vi "Format Event ID.vi"(6 "Channel (Channel A)":enum16{"Channel A", "Channel B"}(ring), 7 "Event Module # (1)":u32=1 min=1 max=14, 9 "Event Type (None)":T1(ring), 10 "Node In":string) -> (1 "Event ID":string, 2 "Node Out":string)   [LabVIEW 2013, in "Keithley 2600 Series.lvlib"]
doc: "This VI will format a string representing an event module's Event Id for use as an input to several of the Advanced Trigger Model VIs."
uses:
  Keithley 2600 Series.lvlib
panel:
  # "(c) 2008 Keithley Instruments, Inc.  ALL RIGHTS RESERVED."
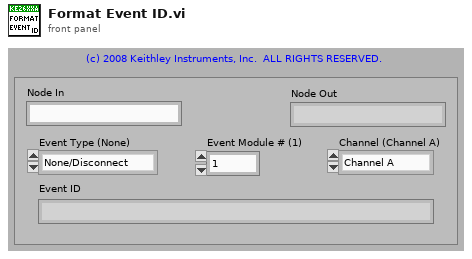
[diagram p1: front panel]
types:
  T1 = enum16{"None/Disconnect", "Digital I/O Trigger", "TSP-Link Trigger", "LAN Trigger", "Blender", "Timer Expired", "Front Panel Trigger", "Software Trigger", "SMU Sweeping", "SMU Armed", "SMU Source Complete", "SMU Measure Complete", "SMU Pulse Complete", "SMU Sweep Complete", "SMU Idle"}
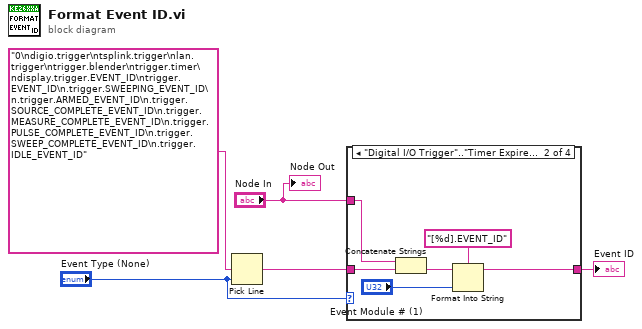
[diagram p0: block diagram]
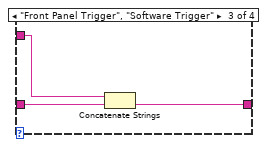
[diagram p3: hidden frame]
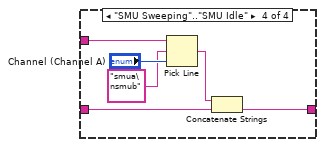
[diagram p4: hidden frame]
diagram:
  n1 = Pick Line(multi-line string="0\ndigio.trigger\ntsplink.trigger\nlan.trigger\ntrigger.blender\ntrigger.timer\ndisplay.trigger.EVENT_ID\ntrigger.EVENT_ID\n.trigger.SWEEPING_EVENT_ID\n.trigger.ARMED_EVENT_ID\n.trigger.SOURCE_COMPLETE_EVENT_ID\n.trigger.MEASURE_COMPLETE_EVENT_ID\n.trigger.PULSE_COMPLETE_EVENT_ID\n.trigger.SWEEP_COMPLETE_EVENT_ID\n.trigger.IDLE_EVENT_ID", line index="Event Type (None)") -> (output string=w3:string)  [unwired: 1 out]
  n2 = case shown="\"Digital I/O Trigger\"..\"Timer Expired\"" "Event Type (None)" {
    tunnel: w3 -> [w6 w9 w14 w19]
    tunnel: [w6 w10 w13 w17] -> w2
    tunnel: "Node In" -> [_ w7 w15 w16]
    frame "None/Disconnect", Default {
    }
    frame "Digital I/O Trigger".."Timer Expired" {
      n3 = Concatenate Strings(w7, w9) -> (w8:string)
      n4 = Format Into String(format string="[%d].EVENT_ID", initial string=w8, "Event Module # (1)") -> (resulting string=w10:string)  [unwired: 1 in, 1 out]
    }
    frame "Front Panel Trigger", "Software Trigger" {
      n5 = Concatenate Strings(w15, w14) -> (w13:string)
    }
    frame "SMU Sweeping".."SMU Idle" {
      n6 = Pick Line(string ("")=w16, multi-line string="smua\nsmub", line index="Channel (Channel A)") -> (output string=w18:string)
      n7 = Concatenate Strings(w18, w19) -> (w17:string)
    }
  }
  "Event ID" <- w2
  "Node Out" <- "Node In"
